vi "Operate.vi"(0 "Arithmetic Operations in":refnum<class "Arithmetic Operations.lvclass">, 11 "error in (no error)":errorcluster) -> (4 "Arithmetic Operations out":refnum<class "Arithmetic Operations.lvclass">, 15 "error out":errorcluster)   [LabVIEW 2020, in "Arithmetic Operations.lvclass"]
uses:
  Arithmetic Operations.lvclass
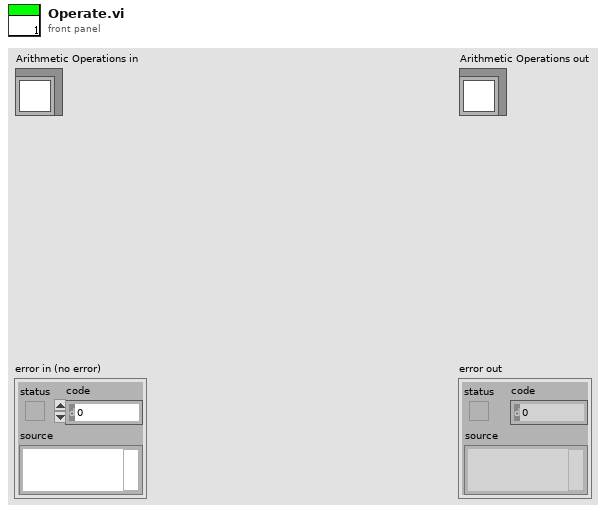
[diagram p1: front panel]
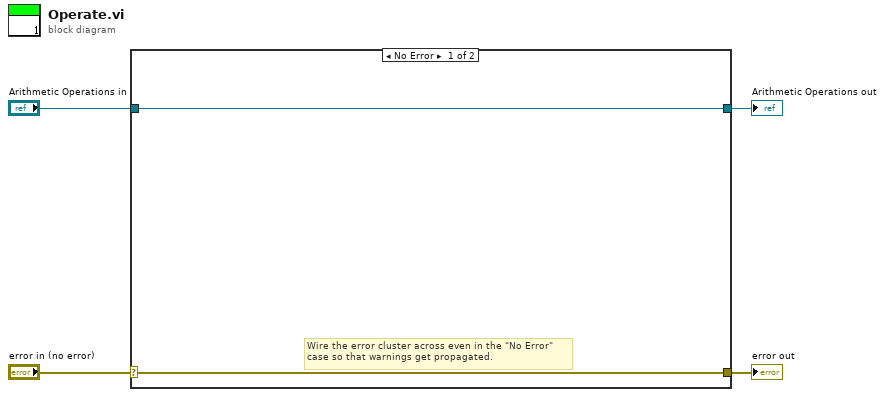
[diagram p0: block diagram]
diagram:
  n1 = case shown="No Error" "error in (no error)" {
    selector: "error in (no error)" -> [w5 w8]
    tunnel: [w5 w8] -> w3
    tunnel: [w6 w7] -> w1
    tunnel: "Arithmetic Operations in" -> [w6 w7]
    frame No Error {
      # "Wire the error cluster across even in the \"No Error\"\ncase so that warnings get propagated."
    }
    frame Error {
    }
  }
  "error out" <- w3
  "Arithmetic Operations out" <- w1
